vi "common_destroy_global_app_event.vi"(8 "error in (no error)":errorcluster) -> (0 "error out":errorcluster)   [LabVIEW 2019]
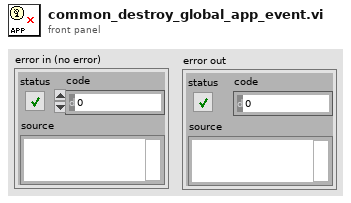
[diagram p1: front panel]
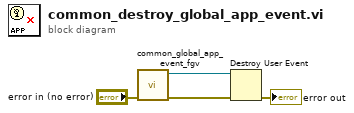
[diagram p0: block diagram]
diagram:
  n1 = call "common_global_app_event_fgv.vi"("error in (no error)"="error in (no error)") -> ("error out"=w3:errorcluster, "app event"=w4:refnum<user-event>)  [unwired: 9 in]
  n2 = Destroy User Event(user event=w4, error in=w3) -> (error out=→"error out":errorcluster)
